vi "FTW-File-GenerateLogFilename.vi"(1 "Date Format":T1=enum."YYYY-MM-DD", 2 "Type":string, 3 "Application":string, 4 "Directory":path) -> (0 "Filepath":path)   [LabVIEW 2013]
uses:
  time/FTW-Time-DisplayFormat-Timestamp.ctl
panel:
  # "Inputs"
  # "Outputs"
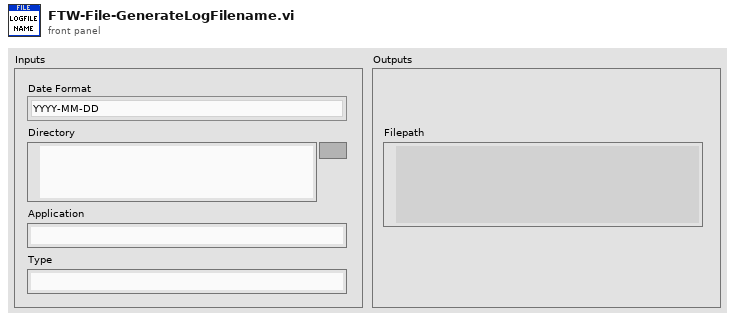
[diagram p1: front panel]
types:
  T1 = typedef "FTW-Time-DisplayFormat-Timestamp.ctl" = enum16{"YYYY-MM-DDT00:00:00.000Z (ISO-8601)", "YYYY-MM-DDT00-00-00Z (Simple ISO-8601)", "YYYY-MM-DD"}
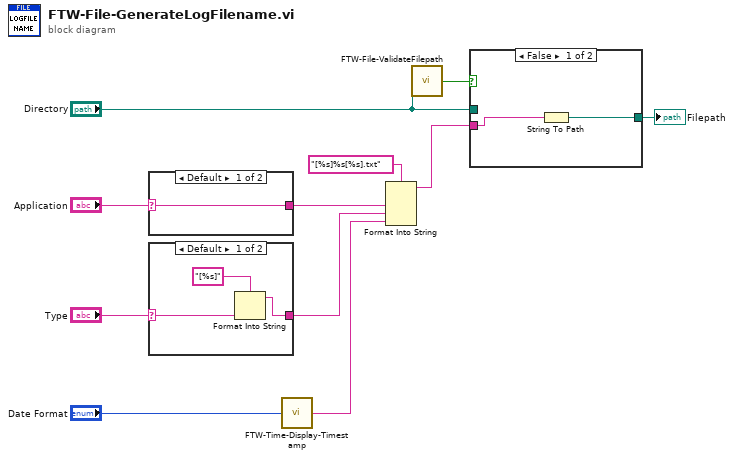
[diagram p0: block diagram]
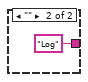
[diagram p2: hidden frame]
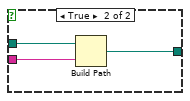
[diagram p4: hidden frame]
diagram:
  n1 = case shown="Default" "Application" {
    selector: "Application" -> [w12 _]
    tunnel: [w12 "Log"] -> w5
    frame Default {
    }
    frame "" {
    }
  }
  n2 = case shown="Default" "Type" {
    selector: "Type" -> [w16 w17]
    tunnel: [w15 w17] -> w7
    frame Default {
      n3 = Format Into String(format string="[%s]", w16) -> (resulting string=w15:string)  [unwired: 2 in, 1 out]
    }
    frame "" {
    }
  }
  n4 = call "FTW-Time-Display-Timestamp.vi"("Format"="Date Format") -> ("Formatted Timestamp"=w2:string)  [unwired: 3 in]
  n5 = Format Into String(format string="[%s]%s[%s].txt", w5, w7, w2) -> (resulting string=w10:string)  [unwired: 2 in, 1 out]
  n6 = call "FTW-File-ValidateFilepath.vi"("Filepath"="Directory") -> ("Valid?"=w3:bool)
  n7 = case shown="False" w3 {
    tunnel: "Directory" -> [_ w22]
    tunnel: w10 -> [w19 w21]
    tunnel: [w18 w20] -> w9
    frame False {
      n8 = String To Path(string=w19) -> (path=w18:path)
    }
    frame True {
      n9 = Build Path(base path=w22, name or relative path=w21) -> (appended path=w20:path)
    }
  }
  "Filepath" <- w9
